vi "Sim to Val.vi"(0 "DH.Modem":T4={"Pin.V"=25.346938775510207, "Pin.mA"=100.0} {"Pin.mA" scale=0.0..200.0; "Pin.V" scale=0.0..36.0}, 5 "DH.PSU":T3={"Pin.V"=600.0, "Pin.mA"=100.0, "24v.V"=25.346938775510207, "24v.A"=2.0, "Temp"=34.0} {"Temp" scale=0.0..200.0; "24v.A" scale=0.0..4.0; "24v.V" scale=0.0..36.0; "Pin.mA" scale=0.0..1000.0; "Pin.V" scale=0.0..1000.0}, 7 "DH.Controller":T2={"Pin.V"=25.346938775510207, "Pin.A"=2.0, "Temp"=0.0, "Acc.X g"=0.0, "Acc.Y g"=0.0, "Acc.Z g"=0.0, "Ain.1 v"=0.0, "Ain.2 v"=0.0, "Ain.3 v"=0.0, "Ain.4 v"=34.0} {"Temp" scale=0.0..200.0; "Ain.4 v" scale=0.0..10.0; "Ain.3 v" scale=0.0..10.0; "Ain.2 v" scale=0.0..10.0; "Ain.1 v" scale=0.0..10.0; "Acc.Z g" scale=-6.0..6.0; "Acc.Y g" scale=-6.0..6.0; "Acc.X g" scale=-6.0..6.0; "Pin.A" scale=0.0..4.0; "Pin.V" scale=0.0..36.0}, 9 "DH.Solonoid driver":T1={"Stroke mm"=25.346938775510207, "Temp"=0.0, "L.cur 1"=0.0, "L.cur 2"=0.0, "L.cur 3"=0.0, "L.cur 4"=0.0, "L.cur 5"=0.0, "L.cur 6"=34.0} {"L.cur 6" scale=0.0..2.0; "L.cur 5" scale=0.0..2.0; "L.cur 4" scale=0.0..2.0; "L.cur 3" scale=0.0..2.0; "L.cur 2" scale=0.0..2.0; "L.cur 1" scale=0.0..2.0; "Stroke mm" scale=0.0..500.0; "Temp" scale=0.0..200.0}, 11 "error in (no error)":errorcluster) -> (6 "Tool Common Analog Variables":dbl[](array[numeric]), 15 "error out":errorcluster)   [LabVIEW 2011]
uses:
  Tool/Stroker/def/Tool Stroker Modem ana.ctl
  Tool/Stroker/def/Tool Stroker PSU ana.ctl
  Tool/Stroker/def/Tool Stroker Controller ana.ctl
  Tool/Stroker/def/Tool Stroker Solonoid ana.ctl
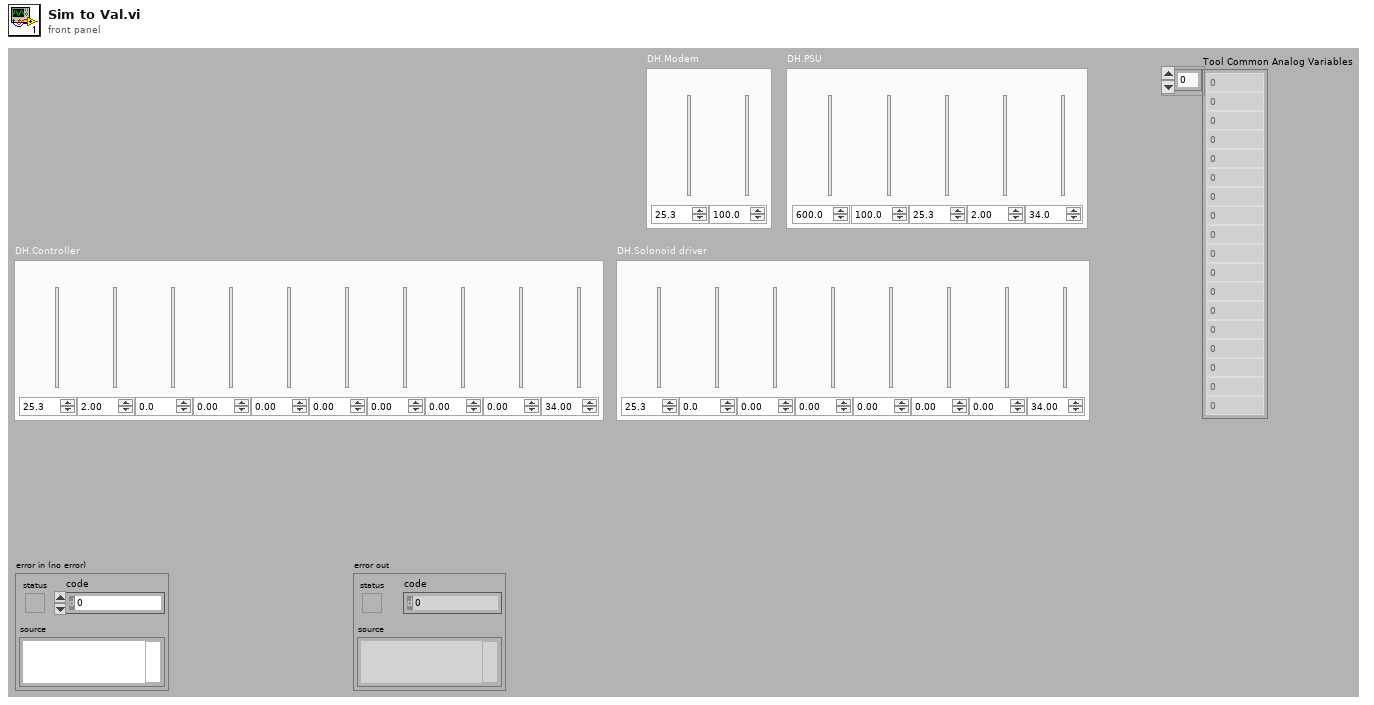
[diagram p1: front panel]
types:
  T1 = typedef "Tool Stroker Solonoid ana.ctl" = cluster{"Stroke mm":dbl, "Temp":dbl, "L.cur 1":dbl, "L.cur 2":dbl, "L.cur 3":dbl, "L.cur 4":dbl, "L.cur 5":dbl, "L.cur 6":dbl}
  T2 = typedef "Tool Stroker Controller ana.ctl" = cluster{"Pin.V":dbl, "Pin.A":dbl, "Temp":dbl, "Acc.X g":dbl, "Acc.Y g":dbl, "Acc.Z g":dbl, "Ain.1 v":dbl, "Ain.2 v":dbl, "Ain.3 v":dbl, "Ain.4 v":dbl}
  T3 = typedef "Tool Stroker PSU ana.ctl" = cluster{"Pin.V":dbl, "Pin.mA":dbl, "24v.V":dbl, "24v.A":dbl, "Temp":dbl}
  T4 = typedef "Tool Stroker Modem ana.ctl" = cluster{"Pin.V":dbl, "Pin.mA":dbl}
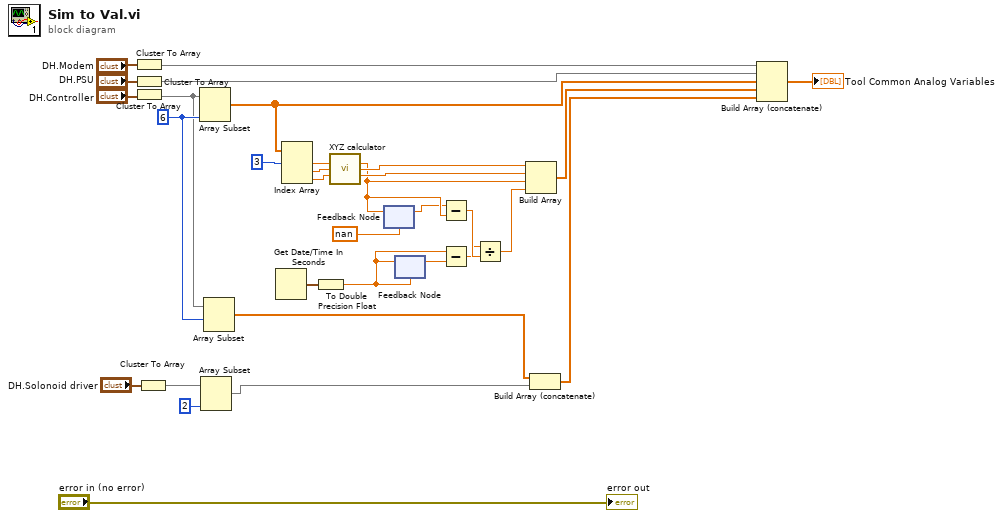
[diagram p0: block diagram]
diagram:
  w27 = 6 ("length")
  n1 = Cluster To Array(cluster="DH.Modem") -> (array=w32:dbl[])
  n2 = Cluster To Array(cluster="DH.PSU") -> (array=w31:dbl[])
  n3 = Cluster To Array(cluster="DH.Controller") -> (array=w26:dbl[])
  n4 = Cluster To Array(cluster="DH.Solonoid driver") -> (array=w16:dbl[])
  n5 = Array Subset(array=w26, length=w27) -> (w22:dbl[])  [unwired: 1 in]
  n6 = Array Subset(array=w16, length=2) -> (w15:dbl[])  [unwired: 1 in]
  n7 = Array Subset(array=w26, index=w27) -> (w24:dbl[])  [unwired: 1 in]
  n8 = Get Date/Time In Seconds() -> (seconds since 1Jan1904=w10:timestamp)
  n9 = Index Array(array=w22, index #1=3 ("index")) -> (element #1=w20:dbl, element #2=w19:dbl, element #3=w18:dbl)  [unwired: 2 in]
  n10 = To Double Precision Float(number=w10) -> (double precision float=w6:dbl)
  n11 = call "XYZ calculator.vi"("X(g)"=w20, "Y(g)"=w19, "Z(g)"=w18) -> ("Angle x-xy"=w9:dbl, "Magnitude XYZ(g)"=w13:dbl, "Angle z-xyz"=w12:dbl)  [unwired: 8 in, 2 out]
  n12 = feedback #1(nan) -> (w8:dbl)
  n13 = feedback-in #1(w9) -> ()
  n14 = feedback #2(w6) -> (w5:dbl)
  n15 = feedback-in #2(w6) -> ()
  n16 = Subtract(x=w8, y=w9) -> (x-y=w7:dbl)
  n17 = Subtract(x=w6, y=w5) -> (x-y=w4:dbl)
  n18 = Divide(x=w4, y=w7) -> (x/y=w3:dbl)
  n19 = Build Array(w13, w12, w9, w3) -> (w17:dbl[])
  n20 = Build Array (concatenate)(w24, w15) -> (w1:dbl[])
  n21 = Build Array (concatenate)(w32, w31, w22, w17, w1) -> (→"Tool Common Analog Variables":dbl[])
  "error out" <- "error in (no error)"
